vi "拆分中文字符串.vi"(8 "error in (no error)":errorcluster caption="错误输入（无错误）", 9 "补足":enum16{"前补", "后补"}(ring)=enum."后补", 10 "索引":i32, 11 "输入字符串":string) -> (0 "error out":errorcluster caption="错误输出", 2 "拆分后":string, 3 "拆分前":string)   [LabVIEW 2016]
uses:
  <vilib>/regexp/Match Regular Expression.xnode
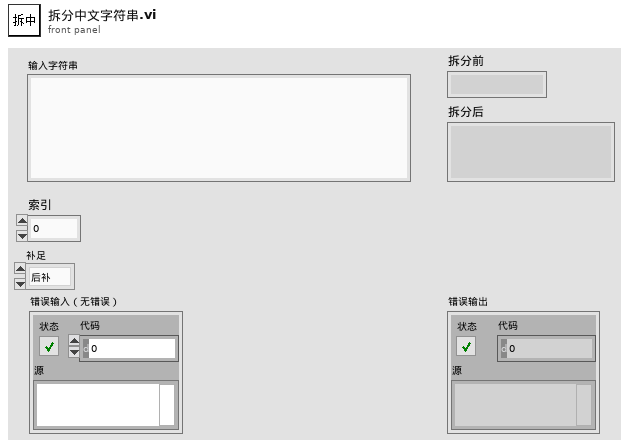
[diagram p1: front panel]
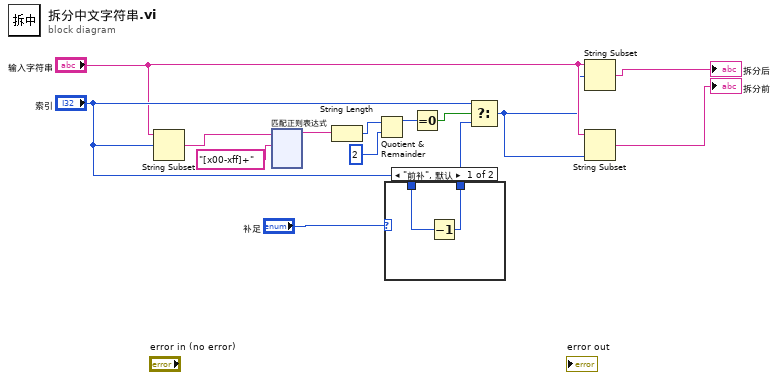
[diagram p0: block diagram]
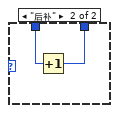
[diagram p2: hidden frame]
diagram:
  n1 = String Subset(string="输入字符串", offset (0)="索引") -> (substring=w5:string)  [unwired: 1 in]
  n2 = xnode "匹配正则表达式"("输入字符串"=w5, "正则表达式"="[x00-xff]+") -> ("匹配之前"=w14:string)  [unwired: 4 in, 4 out]
  n3 = String Length(string=w14) -> (length=w13:i32)
  n4 = Quotient & Remainder(x=w13, y=2) -> (x-y*floor(x/y)=w11:i32)  [unwired: 1 out]
  n5 = case shown="\"前补\", 默认" "补足" {
    tunnel: [w15 w18] -> w9
    tunnel: "索引" -> [w16 w17]
    frame "前补", Default {
      n6 = Decrement(x=w16) -> (x-1=w15:i32)
    }
    frame "后补" {
      n7 = Increment(x=w17) -> (x+1=w18:i32)
    }
  }
  n8 = Equal To 0?(x=w11) -> (x = 0?=w10:bool)
  n9 = Select(t="索引", s=w10, f=w9) -> (s? t:f=w2:i32)
  n10 = String Subset(string="输入字符串", offset (0)=w2) -> (substring=→"拆分后":string)  [unwired: 1 in]
  n11 = String Subset(string="输入字符串", length (rest)=w2) -> (substring=→"拆分前":string)  [unwired: 1 in]
